vi "Read Module Configuration.vi"(8 "error in":errorcluster, 11 "Module Editor Node in":refnum<class "module editor node.lvclass">) -> (0 "error out":errorcluster, 2 "module configuration":refnum<class "TBM module configuration.lvclass">, 3 "Module Editor Node out":refnum<class "module editor node.lvclass">)   [LabVIEW 2013, in "PL Framework Configuration Tool.lvlib" / "module editor node.lvclass"]
uses:
  module editor node.lvclass
  <vilib>/NI/Tag Bus Module Framework/module configuration/TBM module configuration.lvclass
  <vilib>/NI/Configuration Framework/serializable configuration/NISE_CEF_serializable configuration.lvclass
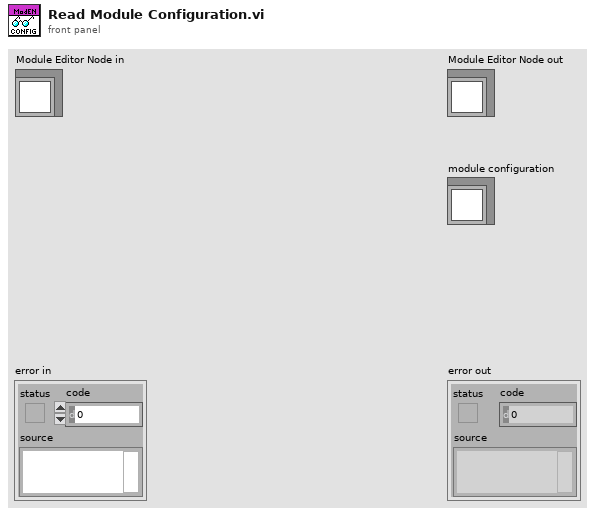
[diagram p1: front panel]
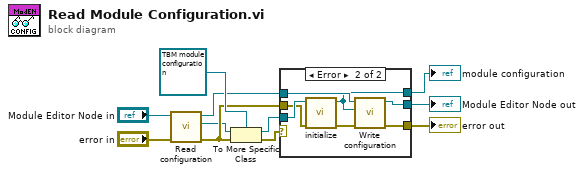
[diagram p0: block diagram]
diagram:
  n1 = call-dynamic "Read configuration.vi"("error in"="error in", "NISE_CEF_serializable node in"="Module Editor Node in") -> ("error out"=w3:errorcluster, "configuration"=w1:refnum<class "NISE_CEF_serializable configuration.lvclass">, "NISE_CEF_serializable node out"=w2:refnum<class "module editor node.lvclass">)  [unwired: 7 in]
  n2 = To More Specific Class(target class=refnum<class "TBM module configuration.lvclass"> refnum ("module configuration"), reference=w1, error in=w3) -> (specific class reference=w10:refnum<class "TBM module configuration.lvclass">, error out=w8:errorcluster)
  n3 = case shown="Error" w8 {
    selector: w8 -> [w12 _]
    tunnel: w10 -> [w14 w21]
    tunnel: [w14 w15] -> w9
    tunnel: w3 -> [_ w20]
    tunnel: w2 -> [w13 w19]
    tunnel: [w13 w18] -> w7
    tunnel: [w12 w17] -> w6
    frame No Error {
    }
    frame Error {
      n4 = call <vilib>:"initialize.vi"("error in"=w20, "configuration in"=w21) -> ("error out"=w16:errorcluster, "configuration out"=w15:refnum<class "TBM module configuration.lvclass">)  [unwired: 7 in, 1 out]
      n5 = call-dynamic "Write configuration.vi"("error in"=w16, "configuration"=w15, "NISE_CEF_serializable node in"=w19) -> ("error out"=w17:errorcluster, "NISE_CEF_serializable node out"=w18:refnum<class "module editor node.lvclass">)  [unwired: 7 in]
    }
  }
  "error out" <- w6
  "Module Editor Node out" <- w7
  "module configuration" <- w9
